vi "Test.vi"   [LabVIEW 2018]
doc: "This VI is called when test mode begins, and will automatically be terminated when it ends. You can add manual or automatic tests and invoke them from the dashboard."
uses:
  Global_Variables/Refnum_Names.vi
  <vilib>/Rock Robotics/WPI/Utilities/WPI_GetSetVariantRefNum.vi
types:
  T1 = typedef "Joystick_Controls.ctl" = cluster{"Pilot Left Joystick X":dbl, "Pilot Left Joystick Y":dbl, "Pilot A Button":bool, "Pilot B Button":bool, "Pilot X Button":bool, "Pilot Y Button":bool, "Pilot Left Bumper":bool, "Pilot Right Bumper":bool, "Pilot View Button":bool, "Pilot Menu Button":bool, "Pilot Left Joystick Press":bool, "Pilot Right Joystick Press":bool, "Pilot Left Trigger":dbl, "Pilot Right Joystick X":dbl, "Pilot Right Joystick Y":dbl, "Pilot Right Trigger":dbl, "Copilot Left Joystick X":dbl, "Copilot Left Joystick Y":dbl, "Copilot A Button":bool, "Copilot B Button":bool, "Copilot X Button":bool, "Copilot Y Button":bool, "Copilot Left Bumper":bool, "Copilot Right Bumper":bool, "Copilot View Button":bool, "Copilot Menu Button":bool, "Copilot Left Joystick Press":bool, "Copilot Right Joystick Press":bool, "Copilot Left Trigger":dbl, "Copilot Right Joystick X":dbl, "Copilot Right Joystick Y":dbl, "Copilot Right Trigger":dbl, "Pilot D-pad North":bool, "Pilot D-pad South":bool, "Pilot D-pad East":bool, "Pilot D-pad West":bool, "Pilot D-pad NE ":bool, "Pilot D-pad SE":bool, "Pilot D-pad SW":bool, "Pilot D-pad NW":bool, "CoPilot D-pad North":bool, "CoPilot D-pad South":bool, "CoPilot D-pad East":bool, "CoPilot D-pad West":bool, "CoPilot D-pad NE":bool, "CoPilot D-pad SE":bool, "CoPilot D-pad SW":bool, "CoPilot D-pad NW":bool, "Pilot Left Trigger Pressed":bool, "Pilot Right Trigger Pressed":bool, "CoPilot Left Trigger Pressed":bool, "CoPilot Right Trigger Pressed":bool}
  T2 = typedef "WPI_JoystickDevRef.ctl" = cluster{"Device":T3}
  T3 = typedef "WPI_JoystickDeviceEnum.ctl" = enum16{"USB 0", "USB 1", "USB 2", "USB 3", "USB 4", "USB 5"}
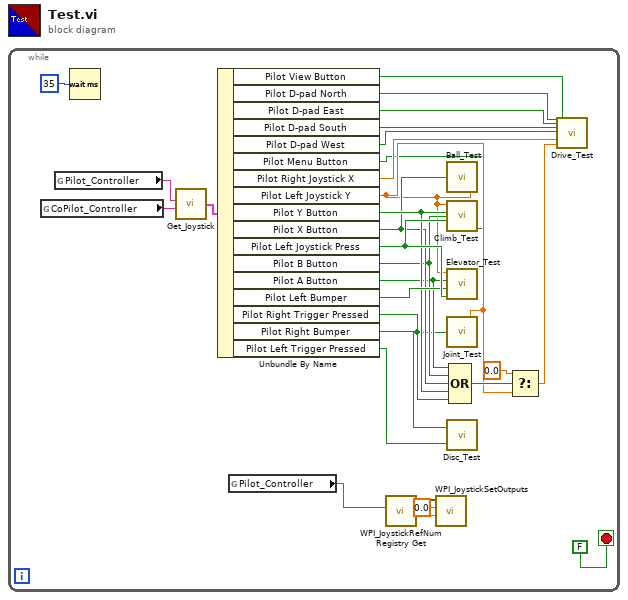
[diagram p0: block diagram]
diagram:
  n1 = while {
    stop <- FALSE stop-if-true
    w3 = sgl 0.0 ("Left Rumble")
    n2 = global read "Refnum_Names.vi" "CoPilot_Controller"() -> (w24:string)
    n3 = global read "Refnum_Names.vi" "Pilot_Controller"() -> (w25:string)
    n4 = Wait (ms)(milliseconds to wait=u32 35) -> ()  [unwired: 1 out]
    n5 = call "Get_Joystick.vi"("Joystick_One"=w25, "Joystick_Two"=w24) -> ("Joystick_Out"=w28:T1)  [unwired: 5 in]
    n6 = Unbundle By Name(w28) -> ("Pilot View Button"=w6:bool, "Pilot D-pad North"=w23:bool, "Pilot D-pad East"=w22:bool, "Pilot D-pad South"=w21:bool, "Pilot D-pad West"=w20:bool, "Pilot Menu Button"=w1:bool, "Pilot Right Joystick X"=w16:dbl, "Pilot Left Joystick Y"=w8:dbl, "Pilot Y Button"=w15:bool, "Pilot X Button"=w14:bool, "Pilot Left Joystick Press"=w19:bool, "Pilot B Button"=w13:bool, "Pilot A Button"=w12:bool, "Pilot Left Bumper"=w18:bool, "Pilot Right Trigger Pressed"=w7:bool, "Pilot Right Bumper"=w17:bool, "Pilot Left Trigger Pressed"=w5:bool)
    n7 = global read "Refnum_Names.vi" "Pilot_Controller"() -> (w2:string)
    n8 = call <vilib>:"WPI_JoystickRefNum Registry Get.vi"("refnum name"=w2) -> ("JoystickDevRef"=w4:T2)  [unwired: 9 in, 1 out]
    n9 = call <vilib>:"WPI_JoystickSetOutputs.vi"("Right Rumble"=w3, "Left Rumble"=w3, "JoystickDevRef"=w4) -> ()  [unwired: 7 in, 2 out]
    n10 = call "Ball_Test.vi"("Left_Joystick_Y"=w8, "X_Button"=w14) -> ()
    n11 = call "Climb_Test.vi"("B_Button"=w13, "Left_Joystick_Y"=w8, "Y_Button"=w15, "Left_Joystick_Press"=w19, "Menu_Button"=w1) -> ()
    n12 = call "Elevator_Test.vi"("Left_Joystick_Press"=w19, "LB_Press"=w18, "A_Button"=w12, "Left_Joystick_Y"=w8) -> ()
    n13 = call "Joint_Test.vi"("Left_Joystick_Y"=w8, "RT_Pressed"=w7) -> ()
    n14 = call "Disc_Test.vi"("LT_Pressed"=w5, "RB_Pressed"=w17) -> ()  [unwired: 1 in]
    n15 = Compound Arithmetic op=OR(w12, w13, w14, w15, w7) -> (w10:bool)
    n16 = Select(t=0.0, s=w10, f=w8) -> (s? t:f=w11:dbl)
    n17 = call "Drive_Test.vi"("Rotate Front Left"=w23, "Rotate Front Right"=w22, "Rotate Back Left"=w21, "Rotate Back Right"=w20, "Test_Joy_X"=w16, "Test_Joy_Y"=w11, "Zero_Gyro"=w6) -> ()  [unwired: 21 in]
  }
